vi "GetForLoopCount.vi"(6 "error in":errorcluster, 9 "ForLoop in":refnum<class "WhileLoop.lvclass">) -> (0 "error out":errorcluster, 3 "ForLoop out":refnum<class "WhileLoop.lvclass">, 4 "count UID":i32)   [LabVIEW 2014]
uses:
  WhileLoop.lvclass
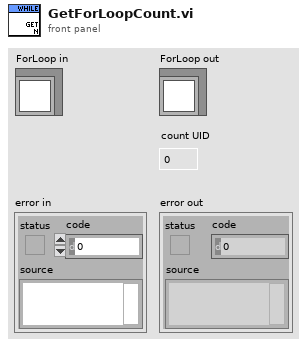
[diagram p1: front panel]
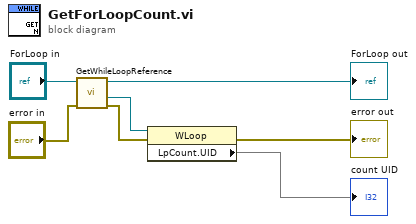
[diagram p0: block diagram]
diagram:
  n1 = call "GetWhileLoopReference.vi"("error in"="error in", "WhileLoop in"="ForLoop in") -> ("error out"=w4:errorcluster, "reference out"=w5:refnum<vi>, "WhileLoop out"=→"ForLoop out":refnum<class "WhileLoop.lvclass">)  [unwired: 7 in]
  n2 = property class="WLoop"(reference=w5, error in=w4) -> (error out=→"error out":errorcluster, "LpCount.UID"=→"count UID")  [unwired: 1 out]
